vi "Inject Fan Controller.vi"(7 "Fan Controller Ref":refnum<data-value>, 8 "error in (no error)":errorcluster, 11 "Start Air Dry in":refnum<class "Start Air Dry.lvclass">) -> (0 "error out":errorcluster, 3 "Start Air Dry out":refnum<class "Start Air Dry.lvclass">)   [LabVIEW 2019, in "Start Air Dry.lvclass"]
uses:
  <vilib>/gpm_packages/@cs/Car-wash/Source/Process Steps/Start Air Dry/Start Air Dry.lvclass
  <vilib>/gpm_packages/@cs/Car-wash/Source/iFan Controller/iFan Controller.lvclass
  <vilib>/gpm_packages/@cs/Car-wash/Source/Process Steps/Start Air Dry/Start Air Dry.lvclass/Start Air Dry.ctl
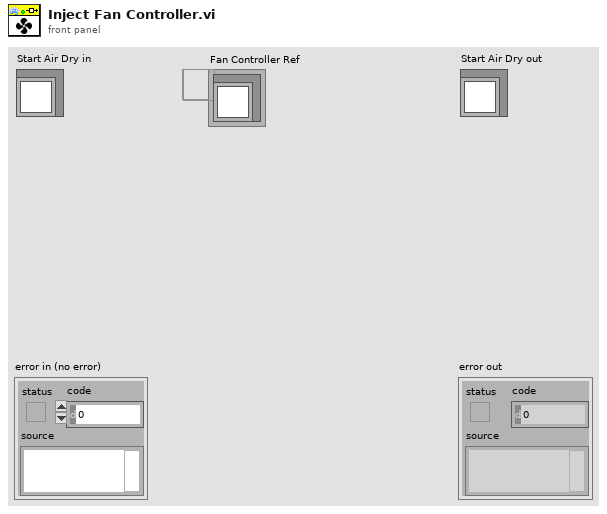
[diagram p1: front panel]
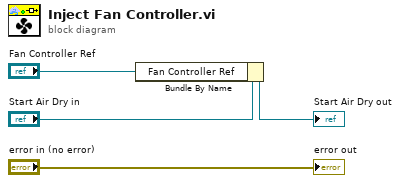
[diagram p0: block diagram]
diagram:
  n1 = Bundle By Name(cluster="Start Air Dry in", "Fan Controller Ref"="Fan Controller Ref") -> (→"Start Air Dry out":refnum<class "Start Air Dry.lvclass">)
  "error out" <- "error in (no error)"
